vi "Execute.vi"(8 "error in (no error)":errorcluster, 9 "write enable":bool=TRUE, 10 "stop":bool, 11 "MB_TCP in":refnum<class "MB_TCP.lvclass">) -> (0 "error out":errorcluster, 2 "stopped":bool, 3 "MB_TCP out":refnum<class "MB_TCP.lvclass">)   [LabVIEW 2019, in "MB_TCP.lvclass"]
uses:
  MB_TCP.lvclass
  MB_TCP_State.ctl
  MB_TCP.lvclass/MB_TCP.ctl
  NI_modbus_upd/TCP/TCP.lvclass/TCP.ctl
  ICPCON Registers/MB ICPCON Registers Write DO.vi
  ICPCON Registers/MB ICPCON Registers Write IR.vi
  ICPCON Registers/MB ICPCON Registers Write DI.vi
  ICPCON Registers/MB ICPCON Registers Write OR.vi
  NI_modbus_upd/TCP/Accessors/Address/Write Address.vi
  NI_modbus_upd/TCP/Accessors/Port/Write Port.vi
  NI_modbus_upd/TCP/Accessors/connect timeout/Write timeouts.vi
  ICPCON Param/MB ICPCON Param Read timeout.vi
  Eth Status/Eth Status Read Error.vi
  Timer Delay/unix time 1ms.vi
  Eth Status/Eth Status.lvlib
  ICPCON Registers/ICPCON Registers.lvlib
  Timer Delay/Timers.lvlib
  ICPCON Param/ICPCON_Param.lvlib
panel:
  out "MB_TCP_State":T1=enum."requests"
  out "t ms":u32
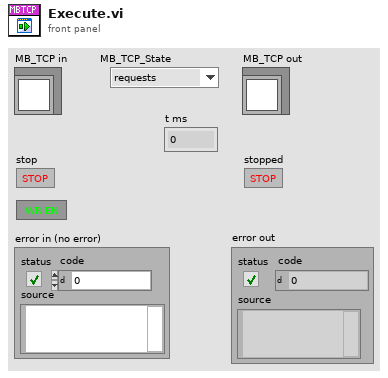
[diagram p1: front panel]
types:
  T1 = typedef "MB_TCP.lvclass/MB_TCP_State.ctl" = enum8{"initialization", "redefine", "standby", "connect", "wait to reconnect", "wait to reset timeout", "configure", "requests", "close connection", "stop"}
  T2 = typedef "ICPCON_Param.lvlib/ICPCON Param.ctl" = cluster{"IP addr":refnum<data-value>, "MVIName":refnum<data-value>, "timeouts":refnum<data-value>, "modified":refnum<data-value>}
  T3 = typedef "ICPCON Registers.lvlib/ICPCON Data.ctl" = cluster{"UTF":refnum<data-value>, "DI":refnum<data-value>, "DW":refnum<data-value>, "DO":refnum<data-value>, "IR":refnum<data-value>, "WR":refnum<data-value>, "OR":refnum<data-value>, "modified":refnum<data-value>}
  T4 = typedef "Eth Status.lvlib/ICPCON Status.ctl" = cluster{"Set_state_com":refnum<data-value>, "start":refnum<data-value>, "WrEn":refnum<data-value>, "errors":refnum<data-value>, "connect":refnum<data-value>, "state":refnum<data-value>}
  T5 = typedef "MB_TCP.lvclass/MB timeouts.ctl" = cluster{"reconn_timeout":i32, "N attempt max":i32, "t_reset_TTL":i32, "period":i32}
  T6 = cluster{"Remote IP Address":string, "Remote Port":u16}
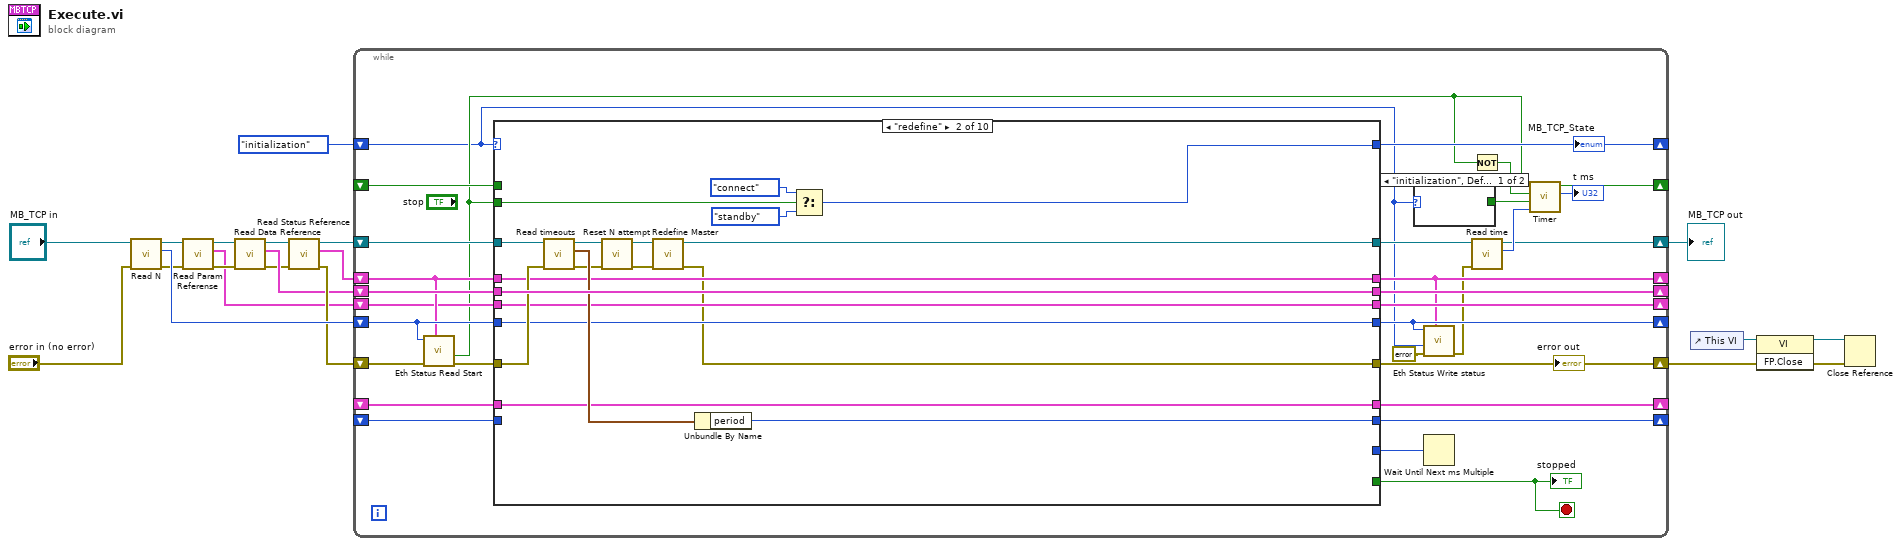
[diagram p0: block diagram]
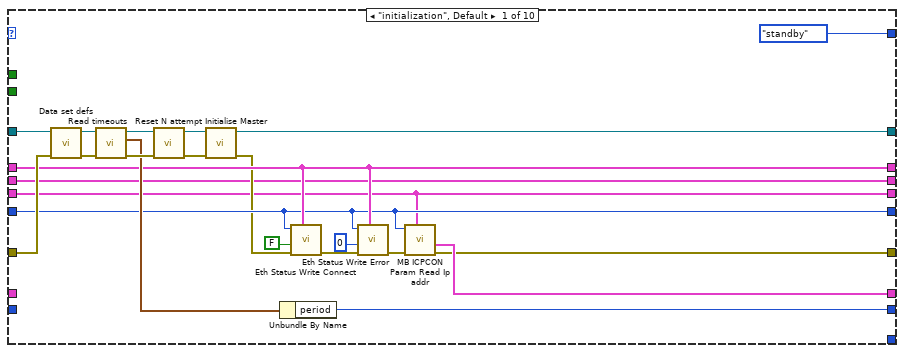
[diagram p2: hidden frame]
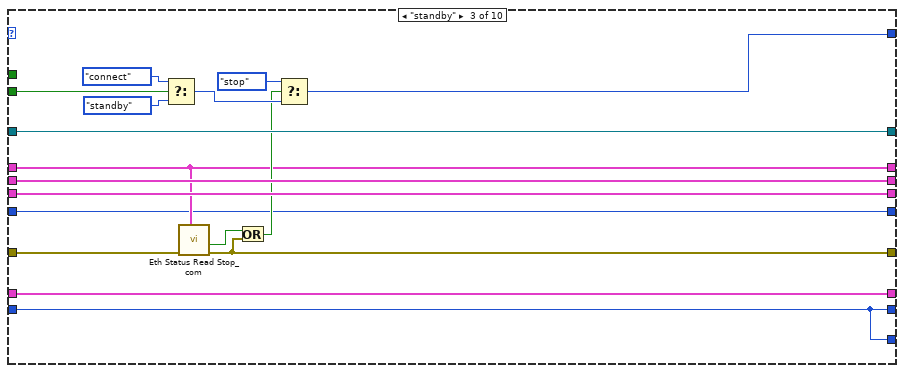
[diagram p3: hidden frame]
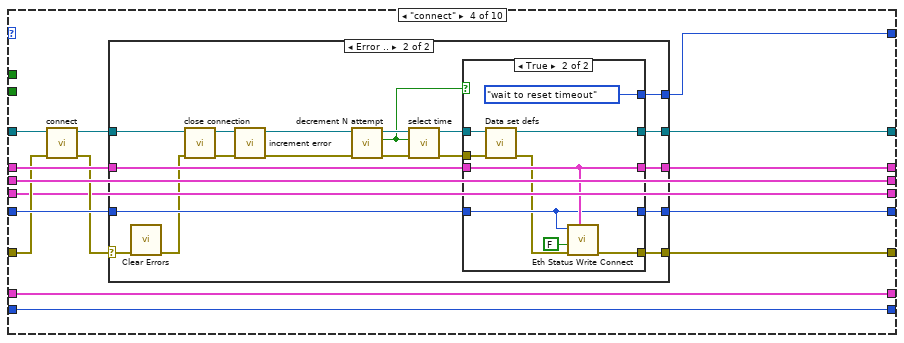
[diagram p4: hidden frame]
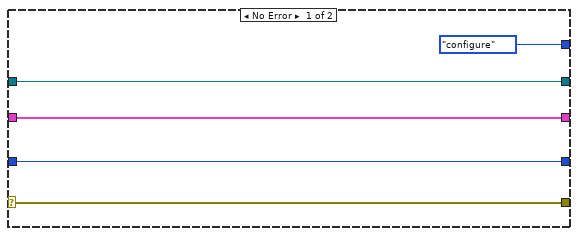
[diagram p5: hidden frame]
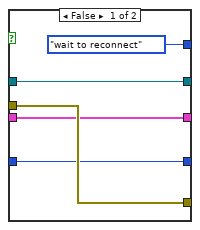
[diagram p6: hidden frame]
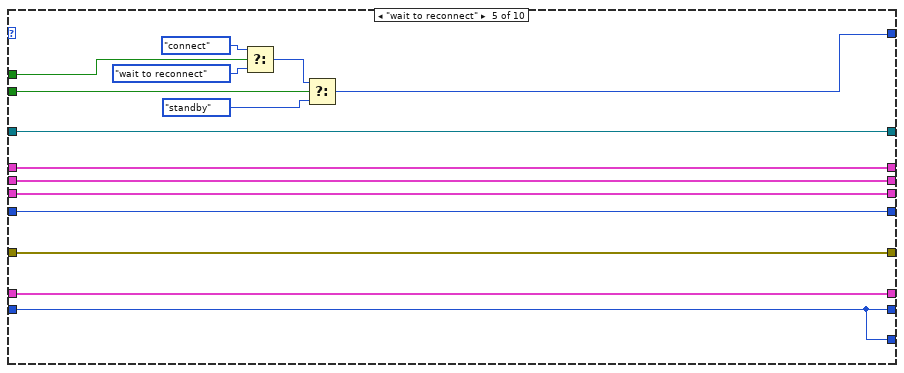
[diagram p7: hidden frame]
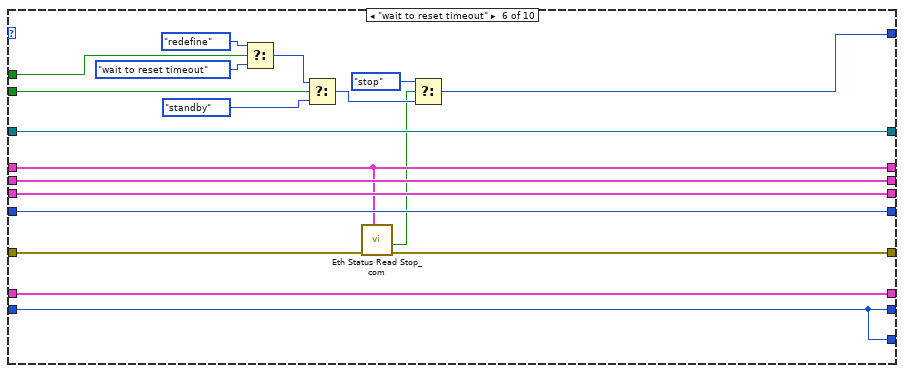
[diagram p8: hidden frame]
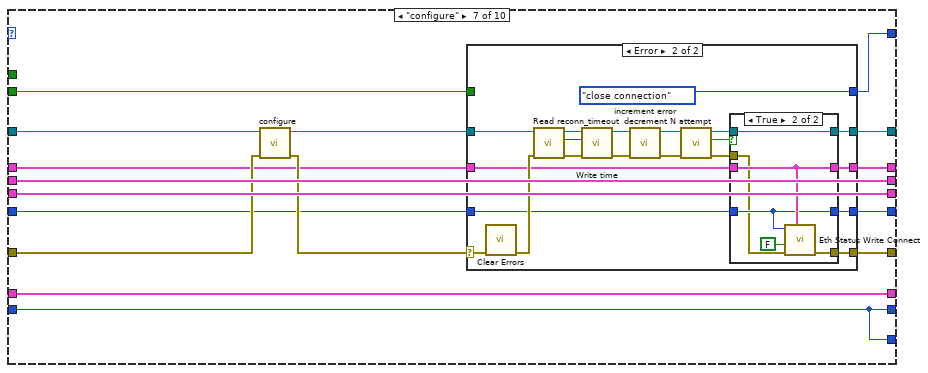
[diagram p9: hidden frame]
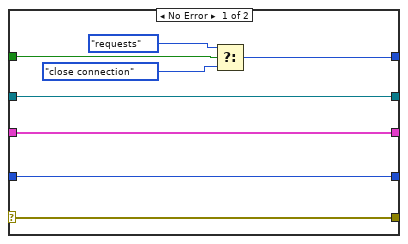
[diagram p10: hidden frame]
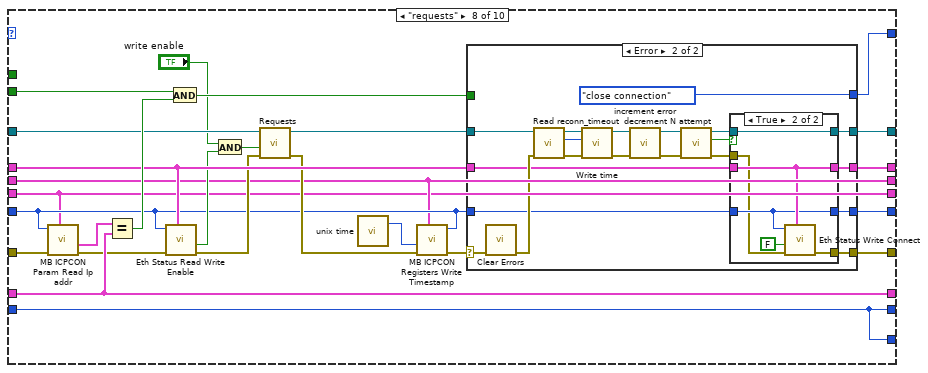
[diagram p12: hidden frame]
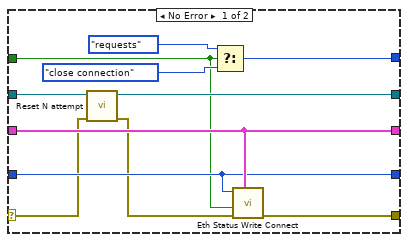
[diagram p13: hidden frame]
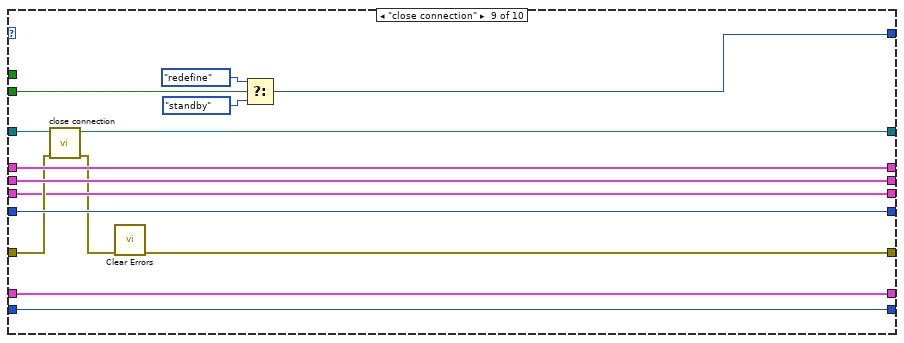
[diagram p15: hidden frame]
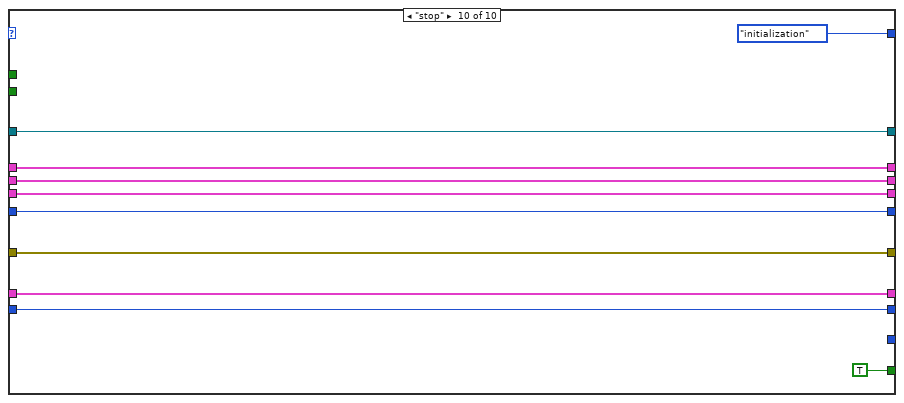
[diagram p16: hidden frame]
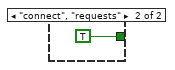
[diagram p17: hidden frame]
diagram:
  n1 = call "Read N.vi"("error in (no error)"="error in (no error)", "MB_TCP in"="MB_TCP in") -> ("error out"=w9:errorcluster, "N"=w15:i32, "MB_TCP out"=w8:refnum<class "MB_TCP.lvclass">)  [unwired: 7 in]
  n2 = call "Read Param Referense.vi"("error in (no error)"=w9, "MB_TCP in"=w8) -> ("error out"=w6:errorcluster, "Param Referense"=w5:T2, "MB_TCP out"=w7:refnum<class "MB_TCP.lvclass">)  [unwired: 7 in]
  n3 = call "Read Data Reference.vi"("error in (no error)"=w6, "MB_TCP in"=w7) -> ("error out"=w10:errorcluster, "Data"=w13:T3, "MB_TCP out"=w11:refnum<class "MB_TCP.lvclass">)  [unwired: 7 in]
  n4 = call "Read Status Reference.vi"("error in (no error)"=w10, "MB_TCP in"=w11) -> ("error out"=w14:errorcluster, "Status"=w16:T4, "MB_TCP out"=w17:refnum<class "MB_TCP.lvclass">)  [unwired: 7 in]
  n5 = while {
    shift-right: [w48] -> _
    shift-left: _ -> [w47]
    shift-right: [w46] -> _
    shift-left: _ -> [w45]
    shift-right: [w44] -> _
    shift-left: w13 -> [w43]
    shift-right: [w30] -> w19
    shift-left: w17 -> [w36]
    shift-right: [w40] -> _
    shift-left: MB_TCP_State."initialization" ("MB_TCP_State") -> [w23]
    shift-right: [w24] -> _
    shift-left: w16 -> [w33]
    shift-right: [w25] -> _
    shift-left: w15 -> [w35]
    shift-right: [w22] -> w3
    shift-left: w14 -> [w26]
    shift-right: [w29] -> _
    shift-left: _ -> [w38]
    shift-right: [w31] -> _
    shift-left: w5 -> [w32]
    stop <- w42 stop-if-true
    n6 = call "Eth Status Read Start.vi"("Status Reference"=w33, "error in (no error)"=w26, "N"=w35) -> ("error out"=w37:errorcluster, "Start"=w27:bool)  [unwired: 7 in]
    n7 = case shown="\"redefine\"" w23 {
      tunnel: w27 -> [_ w92 w109 _ w177 w192 w205 w276 w329 _]
      tunnel: w47 -> [_ _ _ _ w173 w191 _ _ _ _]
      tunnel: [_ _ _ _ _ _ _ _ _ TRUE] -> w42
      tunnel: [w59 w75 w99 w110 w164 w183 w212 w274 w320 w334] -> w46
      tunnel: w45 -> [_ w75 w99 w110 w164 w183 w212 w274 w320 w334]
      tunnel: [w52 w91 w108 w124 w176 w196 w208 w253 w332 w342] -> w44
      tunnel: w43 -> [w52 w91 w108 w124 w176 w196 w208 w253 w332 w342]
      tunnel: w36 -> [w70 w87 w105 w114 w170 w189 w204 w261 w324 w335]
      tunnel: [w53 w77 w105 w123 w170 w189 w211 w269 w322 w335] -> w39
      tunnel: w37 -> [w71 w86 w97 w115 w166 w181 w201 w264 w323 w339]
      tunnel: [MB_TCP_State."standby" ("MB_TCP_State") w88 w102 w122 w169 w184 w210 w268 w328 MB_TCP_State."initialization" ("MB_TCP_State")] -> w40
      tunnel: [w61 w81 w95 w121 w168 w179 w199 w267 w327 w341] -> w24
      tunnel: [w60 w80 w94 w117 w167 w188 w197 w266 w326 w340] -> w25
      tunnel: w33 -> [w61 w81 w95 w120 w168 w179 w200 w263 w327 w341]
      tunnel: w35 -> [w60 w80 w94 w118 w167 w188 w198 w254 w326 w340]
      tunnel: [w57 w74 w93 w119 w166 w180 w209 w265 w318 w339] -> w22
      tunnel: [w72 w84 w98 w116 w163 w182 w206 w251 w325 w338] -> w29
      tunnel: w38 -> [_ _ w98 w116 w163 w182 w206 w251 w325 w338]
      tunnel: w32 -> [w51 w76 w104 w111 w165 w187 w207 w252 w321 w337]
      tunnel: [w51 w76 w104 w111 w165 w187 w207 w252 w321 w337] -> w31
      tunnel: [_ _ w98 _ w163 w182 w206 w251 _ _] -> w28
      frame "initialization", Default {
        n8 = call "Data set defs.vi"("error in (no error)"=w71, "MB_TCP in"=w70) -> ("error out"=w58:errorcluster, "MB_TCP out"=w64:refnum<class "MB_TCP.lvclass">)  [unwired: 8 in]
        n9 = call "Read timeouts.vi"("error in (no error)"=w58, "MB_TCP in"=w64) -> ("error out"=w69:errorcluster, "MB timeouts"=w62:T5, "MB_TCP out"=w63:refnum<class "MB_TCP.lvclass">)  [unwired: 7 in]
        n10 = call "Reset N attempt.vi"("error in (no error)"=w69, "MB_TCP in"=w63) -> ("error out"=w55:errorcluster, "MB_TCP out"=w56:refnum<class "MB_TCP.lvclass">)  [unwired: 8 in]
        n11 = call "Initialise Master.vi"("error in (no error)"=w55, "MB_TCP in"=w56) -> ("error out"=w54:errorcluster, "MB_TCP out"=w53:refnum<class "MB_TCP.lvclass">)  [unwired: 8 in]
        n12 = Unbundle By Name(w62) -> ("period"=w72:i32)
        n13 = call "Eth Status Write Connect.vi"("Status Reference"=w61, "error in (no error)"=w54, "Connect"=FALSE ("connect"), "N"=w60) -> ("error out"=w66:errorcluster)  [unwired: 7 in]
        n14 = call "Eth Status Write Error.vi"("Status Reference"=w61, "error in (no error)"=w66, "Errors"=0 ("N attempt max"), "N"=w60) -> ("error out"=w65:errorcluster)  [unwired: 7 in]
        n15 = call "MB ICPCON Param Read Ip addr.vi"("Param Reference"=w51, "error in (no error)"=w65, "N"=w60) -> ("error out"=w57:errorcluster, "IP address"=w59:T6)  [unwired: 7 in]
      }
      frame "redefine" {
        n16 = call "Read timeouts.vi"("error in (no error)"=w86, "MB_TCP in"=w87) -> ("error out"=w83:errorcluster, "MB timeouts"=w85:T5, "MB_TCP out"=w82:refnum<class "MB_TCP.lvclass">)  [unwired: 7 in]
        n17 = call "Reset N attempt.vi"("error in (no error)"=w83, "MB_TCP in"=w82) -> ("error out"=w78:errorcluster, "MB_TCP out"=w79:refnum<class "MB_TCP.lvclass">)  [unwired: 8 in]
        n18 = call "Redefine Master.vi"("error in (no error)"=w78, "MB_TCP in"=w79) -> ("error out"=w74:errorcluster, "MB_TCP out"=w77:refnum<class "MB_TCP.lvclass">)  [unwired: 8 in]
        n19 = Unbundle By Name(w85) -> ("period"=w84:i32)
        n20 = Select(t=MB_TCP_State."connect" ("MB_TCP_State"), s=w92, f=MB_TCP_State."standby" ("MB_TCP_State")) -> (s? t:f=w88:T1)
      }
      frame "standby" {
        n21 = Select(t=MB_TCP_State."connect" ("MB_TCP_State"), s=w109, f=MB_TCP_State."standby" ("MB_TCP_State")) -> (s? t:f=w101:T1)
        n22 = call "Eth Status Read Stop_com.vi"("Status Reference"=w95, "error in (no error)"=w97) -> ("error out"=w93:errorcluster, "Stop"=w96:bool)  [unwired: 8 in]
        n23 = Or(x=w96, y=w93) -> (x .or. y?=w100:bool)
        n24 = Select(t=MB_TCP_State."stop" ("MB_TCP_State"), s=w100, f=w101) -> (s? t:f=w102:T1)
      }
      frame "connect" {
        n25 = call-dynamic "connect.vi"("error in (no error)"=w115, "MB_TCP in"=w114) -> ("error out"=w112:errorcluster, "MB_TCP out"=w113:refnum<class "MB_TCP.lvclass">)  [unwired: 8 in]
        n26 = case shown="Error .." w112 {
          selector: w112 -> [w127 w132]
          tunnel: w113 -> [w128 w133]
          tunnel: [MB_TCP_State."configure" ("MB_TCP_State") w144] -> w122
          tunnel: [w128 w137] -> w123
          tunnel: [w127 w136] -> w119
          tunnel: w120 -> [w126 w138]
          tunnel: w118 -> [w125 w139]
          tunnel: [w126 w141] -> w121
          tunnel: [w125 w140] -> w117
          frame No Error {
          }
          frame Error {
            n27 = call <vilib>:"Clear Errors.vi"("error in (no error)"=w132) -> ("error out"=w131:errorcluster)  [unwired: 5 in, 1 out]
            n28 = call "close connection.vi"("error in (no error)"=w131, "MB_TCP in"=w133) -> ("error out"=w134:errorcluster, "MB_TCP out"=w135:refnum<class "MB_TCP.lvclass">)  [unwired: 8 in]
            n29 = call "increment error.vi"("error in (no error)"=w134, "MB_TCP in"=w135) -> ("error out"=w130:errorcluster, "MB_TCP out"=w148:refnum<class "MB_TCP.lvclass">)  [unwired: 7 in, 1 out]
            n30 = call "decrement N attempt.vi"("error in (no error)"=w130, "MB_TCP in"=w148) -> ("error out"=w146:errorcluster, "=0"=w145:bool, "MB_TCP out"=w147:refnum<class "MB_TCP.lvclass">)  [unwired: 7 in]
            n31 = call "select time.vi"("error in (no error)"=w146, "N attemt=0"=w145, "MB_TCP in"=w147) -> ("error out"=w142:errorcluster, "MB_TCP out"=w143:refnum<class "MB_TCP.lvclass">)  [unwired: 7 in]
            n32 = case shown="True" w145 {
              tunnel: [MB_TCP_State."wait to reconnect" ("MB_TCP_State") MB_TCP_State."wait to reset timeout" ("MB_TCP_State")] -> w144
              tunnel: w143 -> [w152 w157]
              tunnel: [w152 w155] -> w137
              tunnel: w142 -> [w151 w156]
              tunnel: [w151 w160] -> w136
              tunnel: w138 -> [w150 w159]
              tunnel: w139 -> [w149 w158]
              tunnel: [w150 w159] -> w141
              tunnel: [w149 w158] -> w140
              frame False {
              }
              frame True {
                n33 = call "Data set defs.vi"("error in (no error)"=w156, "MB_TCP in"=w157) -> ("error out"=w154:errorcluster, "MB_TCP out"=w155:refnum<class "MB_TCP.lvclass">)  [unwired: 8 in]
                n34 = call "Eth Status Write Connect.vi"("Status Reference"=w159, "error in (no error)"=w154, "Connect"=FALSE ("f"), "N"=w158) -> ("error out"=w160:errorcluster)  [unwired: 7 in]
              }
            }
          }
        }
      }
      frame "wait to reconnect" {
        n35 = Select(t=MB_TCP_State."connect" ("MB_TCP_State"), s=w173, f=MB_TCP_State."wait to reconnect" ("MB_TCP_State")) -> (s? t:f=w172:T1)
        n36 = Select(t=w172, s=w177, f=MB_TCP_State."standby" ("MB_TCP_State")) -> (s? t:f=w169:T1)
      }
      frame "wait to reset timeout" {
        n37 = Select(t=MB_TCP_State."redefine" ("MB_TCP_State"), s=w191, f=MB_TCP_State."wait to reset timeout" ("MB_TCP_State")) -> (s? t:f=w193:T1)
        n38 = Select(t=w193, s=w192, f=MB_TCP_State."standby" ("MB_TCP_State")) -> (s? t:f=w185:T1)
        n39 = call "Eth Status Read Stop_com.vi"("Status Reference"=w179, "error in (no error)"=w181) -> ("error out"=w180:errorcluster, "Stop"=w178:bool)  [unwired: 8 in]
        n40 = Select(t=MB_TCP_State."stop" ("MB_TCP_State"), s=w178, f=w185) -> (s? t:f=w184:T1)
      }
      frame "configure" {
        n41 = call-dynamic "configure.vi"("error in (no error)"=w201, "MB_TCP in"=w204) -> ("error out"=w202:errorcluster, "MB_TCP out"=w203:refnum<class "MB_TCP.lvclass">)  [unwired: 8 in]
        n42 = case shown="Error" w202 {
          selector: w202 -> [w215 w233]
          tunnel: [w220 MB_TCP_State."close connection" ("MB_TCP_State")] -> w210
          tunnel: w205 -> [w217 _]
          tunnel: [w215 w223] -> w209
          tunnel: w203 -> [w216 w234]
          tunnel: [w216 w224] -> w211
          tunnel: w200 -> [w214 w226]
          tunnel: [w214 w225] -> w199
          tunnel: w198 -> [w213 w222]
          tunnel: [w213 w221] -> w197
          frame No Error {
            n43 = Select(t=MB_TCP_State."requests" ("MB_TCP_State"), s=w217, f=MB_TCP_State."close connection" ("MB_TCP_State")) -> (s? t:f=w220:T1)
          }
          frame Error {
            n44 = call <vilib>:"Clear Errors.vi"("error in (no error)"=w233) -> ("error out"=w232:errorcluster)  [unwired: 5 in, 1 out]
            n45 = call "Read reconn_timeout.vi"("error in (no error)"=w232, "MB_TCP in"=w234) -> ("error out"=w237:errorcluster, "reconn_timeout"=w238:i32, "MB_TCP out"=w239:refnum<class "MB_TCP.lvclass">)  [unwired: 7 in]
            n46 = call "Write time.vi"("error in (no error)"=w237, "time"=w238, "MB_TCP in"=w239) -> ("error out"=w235:errorcluster, "MB_TCP out"=w236:refnum<class "MB_TCP.lvclass">)  [unwired: 7 in]
            n47 = call "increment error.vi"("error in (no error)"=w235, "MB_TCP in"=w236) -> ("error out"=w228:errorcluster, "MB_TCP out"=w227:refnum<class "MB_TCP.lvclass">)  [unwired: 7 in, 1 out]
            n48 = call "decrement N attempt.vi"("error in (no error)"=w228, "MB_TCP in"=w227) -> ("error out"=w229:errorcluster, "=0"=w231:bool, "MB_TCP out"=w230:refnum<class "MB_TCP.lvclass">)  [unwired: 7 in]
            n49 = case shown="True" w231 {
              tunnel: w230 -> [w244 w246]
              tunnel: [w244 w246] -> w224
              tunnel: w229 -> [w243 w245]
              tunnel: [w243 w249] -> w223
              tunnel: w226 -> [w242 w248]
              tunnel: w222 -> [w241 w247]
              tunnel: [w242 w248] -> w225
              tunnel: [w241 w247] -> w221
              frame False {
              }
              frame True {
                n50 = call "Eth Status Write Connect.vi"("Status Reference"=w248, "error in (no error)"=w245, "Connect"=FALSE ("f"), "N"=w247) -> ("error out"=w249:errorcluster)  [unwired: 7 in]
              }
            }
          }
        }
      }
      frame "requests" {
        n51 = call "MB ICPCON Param Read Ip addr.vi"("Param Reference"=w252, "error in (no error)"=w264, "N"=w254) -> ("error out"=w262:errorcluster, "IP address"=w270:T6)  [unwired: 7 in]
        n52 = Equal?(x=w270, y=w274) -> (x = y?=w273:bool)
        n53 = call "Eth Status Read Write Enable.vi"("Status Reference"=w263, "error in (no error)"=w262, "N"=w254) -> ("error out"=w259:errorcluster, "Write Enable"=w257:bool)  [unwired: 7 in]
        n54 = And(x=w276, y=w273) -> (x .and. y?=w275:bool)
        n55 = And(x="write enable", y=w257) -> (x .and. y?=w255:bool)
        n56 = call-dynamic "Requests.vi"("error in (no error)"=w259, "write enable"=w255, "MB_TCP in"=w261) -> ("error out"=w258:errorcluster, "MB_TCP out"=w260:refnum<class "MB_TCP.lvclass">)  [unwired: 7 in]
        n57 = call-poly "unix time.vi"() -> ("unix time (ms)"=w271:u64)  [unwired: 2 in, 1 out]
        n58 = call "MB ICPCON Registers Write Timestamp.vi"("Data Reference"=w253, "error in (no error)"=w258, "UTF"=w271, "N"=w254) -> ("error out"=w272:errorcluster)  [unwired: 7 in]
        n59 = case shown="Error" w272 {
          selector: w272 -> [w281 w300]
          tunnel: [w287 MB_TCP_State."close connection" ("MB_TCP_State")] -> w268
          tunnel: w275 -> [w277 _]
          tunnel: [w280 w290] -> w265
          tunnel: w263 -> [w283 w297]
          tunnel: w260 -> [w284 w301]
          tunnel: [w278 w291] -> w269
          tunnel: [w283 w295] -> w267
          tunnel: w254 -> [w282 w296]
          tunnel: [w282 w294] -> w266
          frame No Error {
            n60 = call "Reset N attempt.vi"("error in (no error)"=w281, "MB_TCP in"=w284) -> ("error out"=w279:errorcluster, "MB_TCP out"=w278:refnum<class "MB_TCP.lvclass">)  [unwired: 8 in]
            n61 = Select(t=MB_TCP_State."requests" ("MB_TCP_State"), s=w277, f=MB_TCP_State."close connection" ("MB_TCP_State")) -> (s? t:f=w287:T1)
            n62 = call "Eth Status Write Connect.vi"("Status Reference"=w283, "error in (no error)"=w279, "Connect"=w277, "N"=w282) -> ("error out"=w280:errorcluster)  [unwired: 7 in]
          }
          frame Error {
            n63 = call <vilib>:"Clear Errors.vi"("error in (no error)"=w300) -> ("error out"=w299:errorcluster)  [unwired: 5 in, 1 out]
            n64 = call "Read reconn_timeout.vi"("error in (no error)"=w299, "MB_TCP in"=w301) -> ("error out"=w304:errorcluster, "reconn_timeout"=w305:i32, "MB_TCP out"=w306:refnum<class "MB_TCP.lvclass">)  [unwired: 7 in]
            n65 = call "Write time.vi"("error in (no error)"=w304, "time"=w305, "MB_TCP in"=w306) -> ("error out"=w302:errorcluster, "MB_TCP out"=w303:refnum<class "MB_TCP.lvclass">)  [unwired: 7 in]
            n66 = call "increment error.vi"("error in (no error)"=w302, "MB_TCP in"=w303) -> ("error out"=w288:errorcluster, "MB_TCP out"=w293:refnum<class "MB_TCP.lvclass">)  [unwired: 7 in, 1 out]
            n67 = call "decrement N attempt.vi"("error in (no error)"=w288, "MB_TCP in"=w293) -> ("error out"=w289:errorcluster, "=0"=w298:bool, "MB_TCP out"=w292:refnum<class "MB_TCP.lvclass">)  [unwired: 7 in]
            n68 = case shown="True" w298 {
              tunnel: w292 -> [w311 w313]
              tunnel: [w311 w313] -> w291
              tunnel: w289 -> [w310 w312]
              tunnel: [w310 w316] -> w290
              tunnel: w297 -> [w309 w315]
              tunnel: w296 -> [w308 w314]
              tunnel: [w309 w315] -> w295
              tunnel: [w308 w314] -> w294
              frame False {
              }
              frame True {
                n69 = call "Eth Status Write Connect.vi"("Status Reference"=w315, "error in (no error)"=w312, "Connect"=FALSE ("f"), "N"=w314) -> ("error out"=w316:errorcluster)  [unwired: 7 in]
              }
            }
          }
        }
      }
      frame "close connection" {
        n70 = call "close connection.vi"("error in (no error)"=w323, "MB_TCP in"=w324) -> ("error out"=w319:errorcluster, "MB_TCP out"=w322:refnum<class "MB_TCP.lvclass">)  [unwired: 8 in]
        n71 = call <vilib>:"Clear Errors.vi"("error in (no error)"=w319) -> ("error out"=w318:errorcluster)  [unwired: 5 in, 1 out]
        n72 = Select(t=MB_TCP_State."redefine" ("MB_TCP_State"), s=w329, f=MB_TCP_State."standby" ("MB_TCP_State")) -> (s? t:f=w328:T1)
      }
      frame "stop" {
      }
    }
    "stopped" <- w42
    "error out" <- w22
    "MB_TCP_State" <- w40
    n73 = case shown="\"initialization\", Default" w23 {
      tunnel: [_ TRUE] -> w49
      frame "initialization", Default {
      }
      frame "connect", "requests" {
      }
    }
    n74 = call "Eth Status Write status.vi"("Status Reference"=w24, "error in (no error)"=errorcluster {"status"=FALSE, "code"=0, "source"=""}, "status"=w23, "N"=w25) -> ("error out"=w20:errorcluster)  [unwired: 7 in]
    n75 = Wait Until Next ms Multiple(millisecond multiple=w28) -> ()  [unwired: 1 out]
    n76 = Not(x=w27) -> (.not. x?=w50:bool)
    n77 = call "Read time.vi"("error in (no error)"=w20, "MB_TCP in"=w39) -> ("time"=w41:i32, "MB_TCP out"=w30:refnum<class "MB_TCP.lvclass">)  [unwired: 7 in, 1 out]
    n78 = call "Timer.vi"("ms"=w41, "Load (F)"=w49, "Reset (F)"=w50, "Start (T)"=w27) -> ("t ms"=→"t ms":u32, "End"=w48:bool)  [unwired: 5 in]
  }
  "MB_TCP out" <- w19
  n79 = control-ref of="This VI"() -> (w2:refnum<vi>)
  n80 = invoke class="VI" method="FP.Close"(reference=w2) -> (reference out=w1:refnum<vi>)  [unwired: 2 in, 2 out]
  n81 = Close Reference(reference=w1, error in (no error)=w3) -> ()  [unwired: 1 out]
